vi "Calculate  BG Property.vi"(4 "Flip?":bool, 6 "Radius Array":i16[](array[numeric]), 9 "Gird Color":cluster{"Major Color":u32, "Minor Color":u32}, 10 "Plot Area Bounds":T4, 11 "Zero Point Coords":T3) -> (1 "BG Image Property":T1)   [LabVIEW 2017, in "2D Compass.lvclass"]
uses:
  <vilib>/Math Plots/2D Math Plots/2D Compass/2D Compass/2D Compass.lvclass
  <vilib>/Utility/miscctls.llb/LVPoint32TypeDef.ctl
  <vilib>/Math Plots/2D Math Plots/2D Compass/2D Compass/Typedef/BG Image Property.ctl
  <vilib>/Utility/miscctls.llb/LVRectTypeDef.ctl
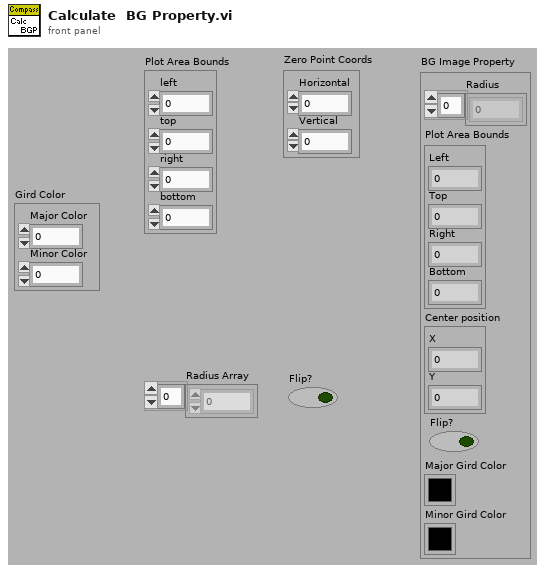
[diagram p1: front panel]
types:
  T1 = typedef "2D Compass.lvclass/BG Image Property.ctl" = cluster{"Radius":i16[], "Plot Area Bounds":T2, "Center position":cluster{"X":i16, "Y":i16}, "Flip?":bool, "Major Gird Color":u32, "Minor Gird Color":u32}
  T2 = typedef "LVRectTypeDef.ctl" = cluster{"Left":i16, "Top":i16, "Right":i16, "Bottom":i16}
  T3 = typedef "LVPoint32TypeDef.ctl" = cluster{"Horizontal":i32, "Vertical":i32}
  T4 = cluster{"left":i32, "top":i32, "right":i32, "bottom":i32}
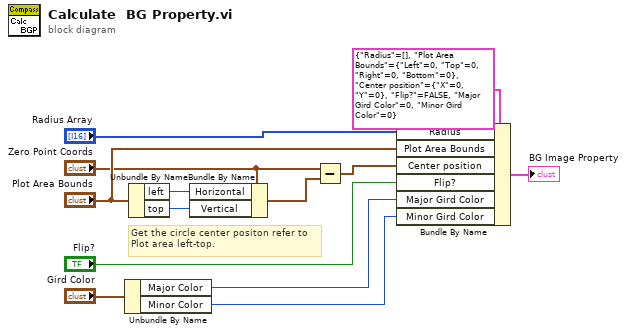
[diagram p0: block diagram]
diagram:
  # "Get the circle center positon refer to\nPlot area left-top."
  n1 = Unbundle By Name("Gird Color") -> ("Major Color"=w2:u32, "Minor Color"=w1:u32)
  n2 = Unbundle By Name("Plot Area Bounds") -> ("left"=w5:i32, "top"=w6:i32)
  n3 = Bundle By Name(cluster="Zero Point Coords", "Horizontal"=w5, "Vertical"=w6) -> (w7:T3)
  n4 = Subtract(x="Zero Point Coords", y=w7) -> (x-y=w8:T3)
  n5 = Bundle By Name(cluster=T1 {"Radius"=[], "Plot Area Bounds"={"Left"=0, "Top"=0, "Right"=0, "Bottom"=0}, "Center position"={"X"=0, "Y"=0}, "Flip?"=FALSE, "Major Gird Color"=0, "Minor Gird Color"=0} ("BG Image Property"), "Radius"="Radius Array", "Plot Area Bounds"="Plot Area Bounds", "Center position"=w8, "Flip?"="Flip?", "Major Gird Color"=w2, "Minor Gird Color"=w1) -> (→"BG Image Property":T1)
